vi "Read Enable.vi"(8 "error in (no error)":errorcluster, 11 "ProjectLoader in":refnum<class "ProjectLoader.lvclass">) -> (0 "error out":errorcluster, 2 "Enable":bool, 3 "ProjectLoader out":refnum<class "ProjectLoader.lvclass">)   [LabVIEW 2015, in "ProjectLoader.lvclass"]
uses:
  ProjectLoader.lvclass
  ProjectLoader.lvclass/ProjectLoader.ctl
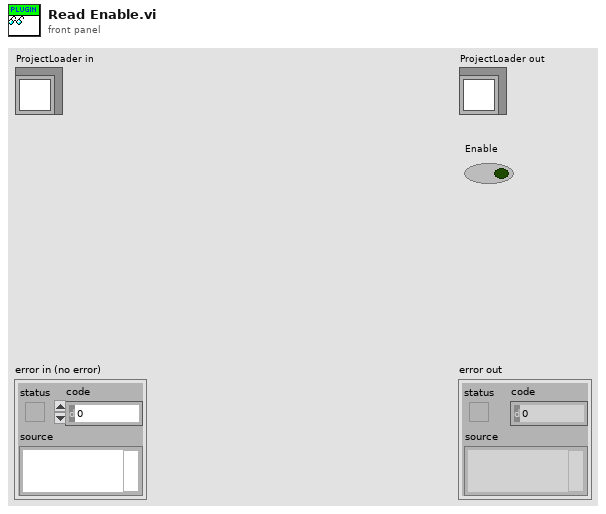
[diagram p1: front panel]
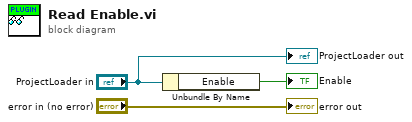
[diagram p0: block diagram]
diagram:
  n1 = Unbundle By Name("ProjectLoader in") -> ("Enable"=→"Enable":bool)
  "error out" <- "error in (no error)"
  "ProjectLoader out" <- "ProjectLoader in"
